vi "2 Bit Increment COunter.vi"(7 "Increment":bool) -> (8 "Counter Value":fxp<+,2,2>)   [LabVIEW 2012]
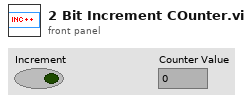
[diagram p1: front panel]
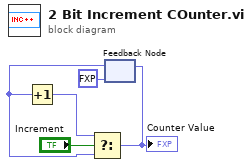
[diagram p0: block diagram]
diagram:
  n1 = feedback #1(fxp<+,2,2> 0.0) -> (w2:fxp<+,2,2>)
  n2 = Increment(x=w2) -> (x+1=w4:fxp<+,2,2>)
  n3 = Select(t=w4, s="Increment", f=w2) -> (s? t:f=w1:fxp<+,2,2>)
  "Counter Value" <- w1
  n4 = feedback-in #1(w1) -> ()
